vi "Take time & dt from path.vi"(0 "Array":dbl[][](array[numeric]), 1 "path":path) -> (2 "Start data 1":string, 3 "Stop data 1":string, 4 "Delta T (s)":dbl, 5 "dt id (ms)":dbl)   [LabVIEW 2012]
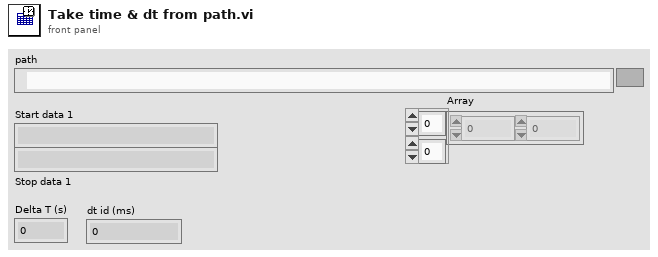
[diagram p1: front panel]
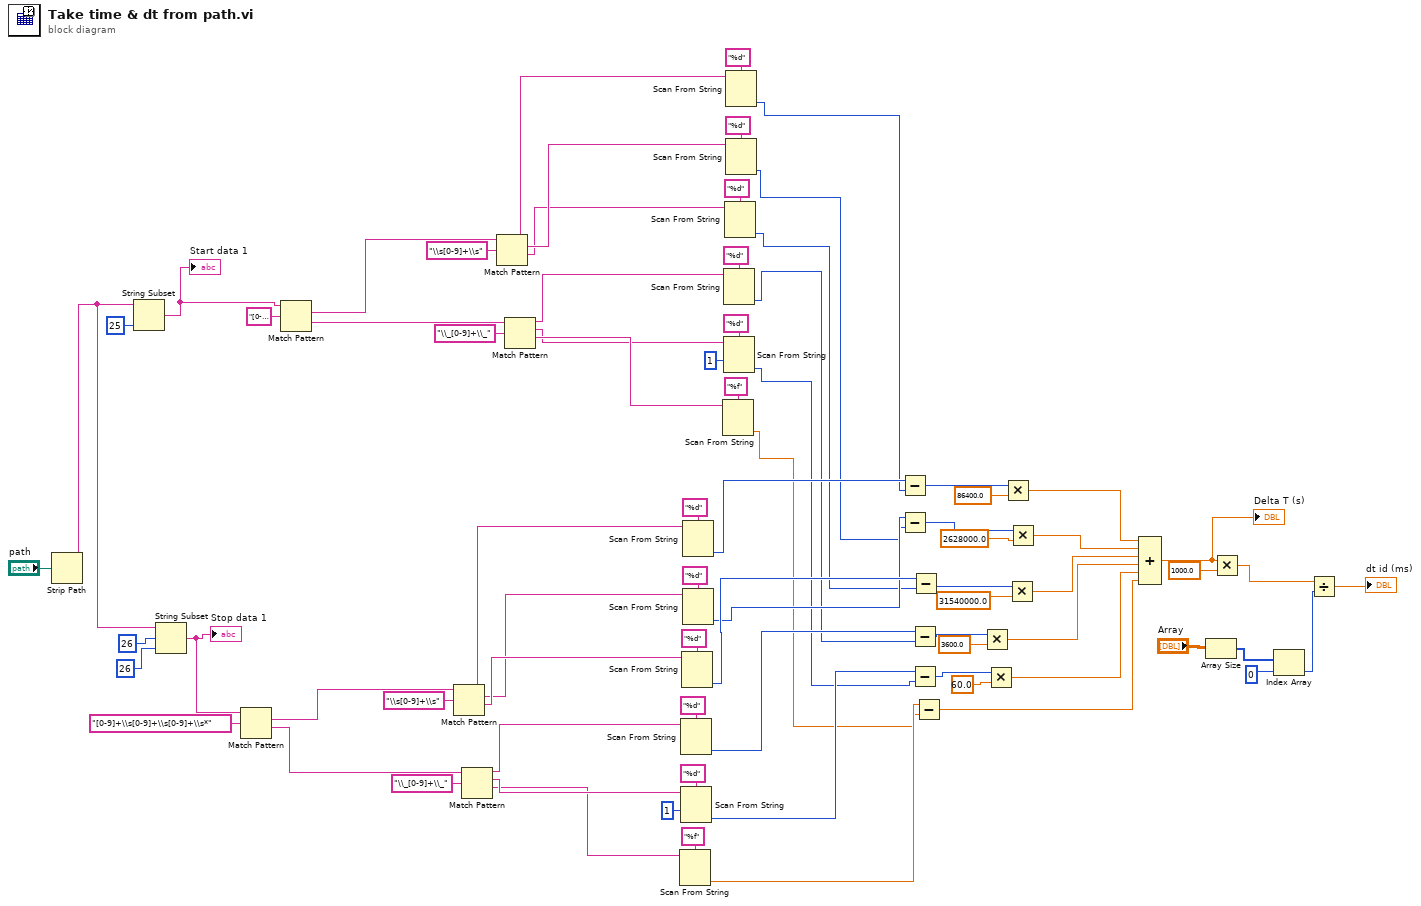
[diagram p0: block diagram]
diagram:
  n1 = Strip Path(path="path") -> (name=w76:string)  [unwired: 1 out]
  n2 = String Subset(string=w76, length (rest)=25 ("length (rest)")) -> (substring=w71:string)  [unwired: 1 in]
  "Start data 1" <- w71
  n3 = String Subset(string=w76, offset (0)=26 ("length (rest)"), length (rest)=26 ("length (rest)")) -> (substring=w74:string)
  "Stop data 1" <- w74
  n4 = Match Pattern(string=w74, regular expression="[0-9]+\\s[0-9]+\\s[0-9]+\\s*") -> (match substring=w70:string, after substring=w64:string)  [unwired: 1 in, 2 out]
  n5 = Match Pattern(string=w71, regular expression="[0-9]+\\s[0-9]+\\s[0-9]+\\s*") -> (match substring=w38:string, after substring=w37:string)  [unwired: 1 in, 2 out]
  n6 = Match Pattern(string=w70, regular expression="\\s[0-9]+\\s") -> (before substring=w54:string, match substring=w55:string, after substring=w56:string)  [unwired: 1 in, 1 out]
  n7 = Match Pattern(string=w64, regular expression="\\_[0-9]+\\_") -> (before substring=w60:string, match substring=w65:string, after substring=w61:string)  [unwired: 1 in, 1 out]
  n8 = Match Pattern(string=w38, regular expression="\\s[0-9]+\\s") -> (before substring=w53:string, match substring=w52:string, after substring=w51:string)  [unwired: 1 in, 1 out]
  n9 = Match Pattern(string=w37, regular expression="\\_[0-9]+\\_") -> (before substring=w47:string, match substring=w43:string, after substring=w46:string)  [unwired: 1 in, 1 out]
  n10 = Scan From String(format string="%f", input string=w61) -> (output 1=w36:dbl)  [unwired: 3 in, 3 out]
  n11 = Scan From String(format string="%d", input string=w60) -> (output 1=w34:i32)  [unwired: 3 in, 3 out]
  n12 = Scan From String(format string="%d", input string=w65, initial scan location=u32 1) -> (output 1=w35:i32)  [unwired: 2 in, 3 out]
  n13 = Scan From String(format string="%d", input string=w56) -> (output 1=w33:i32)  [unwired: 3 in, 3 out]
  n14 = Scan From String(format string="%d", input string=w54) -> (output 1=w31:i32)  [unwired: 3 in, 3 out]
  n15 = Scan From String(format string="%d", input string=w55) -> (output 1=w32:i32)  [unwired: 3 in, 3 out]
  n16 = Scan From String(format string="%f", input string=w46) -> (output 1=w30:dbl)  [unwired: 3 in, 3 out]
  n17 = Scan From String(format string="%d", input string=w47) -> (output 1=w28:i32)  [unwired: 3 in, 3 out]
  n18 = Scan From String(format string="%d", input string=w43, initial scan location=u32 1) -> (output 1=w29:i32)  [unwired: 2 in, 3 out]
  n19 = Scan From String(format string="%d", input string=w51) -> (output 1=w27:i32)  [unwired: 3 in, 3 out]
  n20 = Scan From String(format string="%d", input string=w53) -> (output 1=w25:i32)  [unwired: 3 in, 3 out]
  n21 = Scan From String(format string="%d", input string=w52) -> (output 1=w26:i32)  [unwired: 3 in, 3 out]
  n22 = Subtract(x=w31, y=w25) -> (x-y=w15:i32)
  n23 = Subtract(x=w32, y=w26) -> (x-y=w16:i32)
  n24 = Subtract(x=w34, y=w28) -> (x-y=w21:i32)
  n25 = Subtract(x=w35, y=w29) -> (x-y=w24:i32)
  n26 = Subtract(x=w33, y=w27) -> (x-y=w17:i32)
  n27 = Subtract(x=w36, y=w30) -> (x-y=w9:dbl)
  n28 = Multiply(x=w21, y=3600.0) -> (x*y=w11:dbl)
  n29 = Multiply(x=w24, y=60.0) -> (x*y=w10:dbl)
  n30 = Multiply(x=w15, y=86400.0) -> (x*y=w14:dbl)
  n31 = Multiply(x=w17, y=31540000.0) -> (x*y=w12:dbl)
  n32 = Multiply(x=w16, y=2628000.0) -> (x*y=w13:dbl)
  n33 = Compound Arithmetic op=ADD(w14, w13, w12, w11, w10, w9) -> (w1:dbl)
  "Delta T (s)" <- w1
  n34 = Array Size(array="Array") -> (size(s)=w3:i32[])
  n35 = Multiply(x=w1, y=1000.0) -> (x*y=w6:dbl)
  n36 = Index Array(array=w3, index=0) -> (element=w5:i32)
  n37 = Divide(x=w6, y=w5) -> (x/y=→"dt id (ms)":dbl)
